vi "Get cursor position.vi"(4 "error out":errorcluster, 5 "input main cluster":T1) -> (0 "error out":errorcluster, 1 "output main cluster":T1, 3 "Cursor.Cursor Position":dbl[](array[numeric]))   [LabVIEW 2009]
uses:
  Main_cluster.ctl
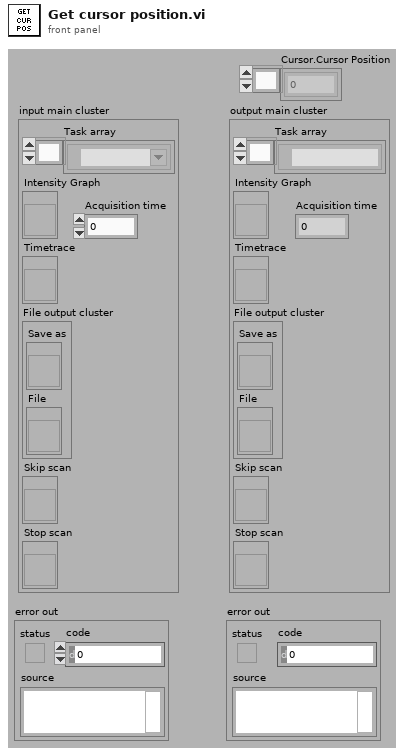
[diagram p1: front panel]
types:
  T1 = typedef "Main_cluster.ctl" = cluster{"Task array":refnum<k21>[], "Intensity Graph":refnum<vi>, "Timetrace":refnum<vi>, "File output cluster":cluster{"Save as":refnum<vi>, "File":refnum<vi>}, "Skip scan":refnum<vi>, "Stop scan":refnum<vi>, "Acquisition time":dbl}
  T2 = typedef "LVPointDoubleTypeDef.ctl" = cluster{"Cursor X":dbl, "Cursor Y":dbl}
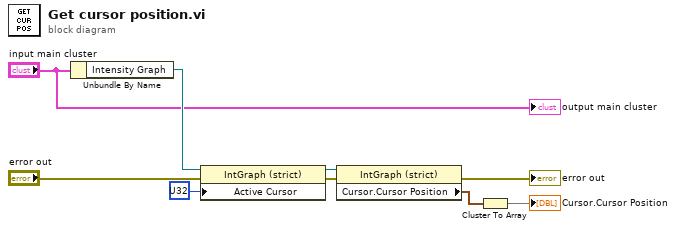
[diagram p0: block diagram]
diagram:
  n1 = Unbundle By Name("input main cluster") -> ("Intensity Graph"=w3:refnum<vi>)
  n2 = property on="Property Node" class="IntGraph (strict)"(reference=w3, error in="error out", "Active Cursor"=u32 ?) -> (reference out=w2:refnum<vi>, error out=w9:errorcluster)
  n3 = property on="Property Node" class="IntGraph (strict)"(reference=w2, error in=w9) -> (error out=→"error out":errorcluster, "Cursor.Cursor Position"=w5:T2)  [unwired: 1 out]
  n4 = Cluster To Array(cluster=w5) -> (array=→"Cursor.Cursor Position":dbl[])
  "output main cluster" <- "input main cluster"
